vi "LCAIO Set Output Sw Scaling Param.vi"(8 "error in (no error)":errorcluster caption="Fehler (Eingang, kein Fehler)", 9 "Scaling Offset":dbl, 10 "Scaling Factor":dbl, 11 "Output Channel Handle":i64) -> (0 "error out":errorcluster caption="Fehler (Ausgang)")   [LabVIEW 2021, in "labbCAN_AnalogIO_API.lvlib"]
doc: "LCAIO_Func long LCAIO_CALL LCAIO_SetOutputSwScalingParam(dev_hdl OutChanHdl,\n double ScalingFactor,\n double ScalingOffset);"
uses:
  labbCAN_AnalogIO_API.lvlib
  labbCAN_AnalogIO_API.dll
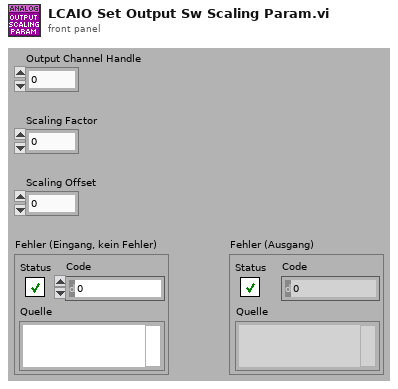
[diagram p1: front panel]
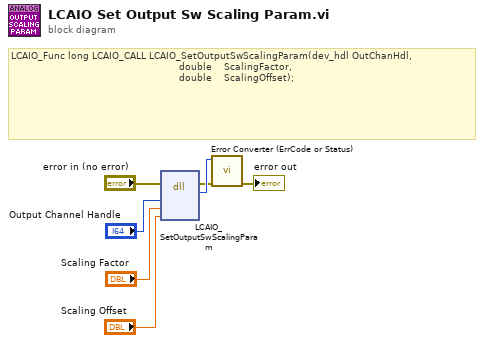
[diagram p0: block diagram]
diagram:
  # "LCAIO_Func long LCAIO_CALL LCAIO_SetOutputSwScalingParam(dev_hdl OutChanHdl,\n                                                        double    ScalingFactor,\n                                                        double    ScalingOffset);"
  n1 = dll-call lib="C:/Users/olaja/AppData/Local/CETONI_SDK/labbCAN_AnalogIO_API.*" fn="LCAIO_SetOutputSwScalingParam"(error in="error in (no error)", "Output Channel Handle"="Output Channel Handle", "Scaling Factor"="Scaling Factor", "Scaling Offset"="Scaling Offset") -> (error out=w2:errorcluster, "Rückgabetyp"=w3:i32)  [unwired: 5 in, 1 out]
  n2 = call "Error Converter (ErrCode or Status).vi"("error in (no error)"=w2, "error code"=w3) -> ("error out"=→"error out":errorcluster)  [unwired: 9 in]
